vi "cast_to_32_bit.vi"(8 "input valid":bool=TRUE, 11 "x":fxp<+/-,64,48>) -> (0 "output valid":bool, 3 "y":fxp<+/-,32,14>)   [LabVIEW 2018]
uses:
  <vilib>/rvi/FXPMathLib/FxpConvert/subVIs/nifxpmath_Convert_SimConfig.ctl
  <vilib>/fxp/LVFixedPointQuantizationPolicyTypeDef.ctl
  <vilib>/fxp/LVFixedPointOverflowPolicyTypeDef.ctl
  <vilib>/rvi/FXPMathLib/FxpConvert/simVIs/DllFxpConvertTemp_sub.vi
  <vilib>/rvi/FXPMathLib/FxpInterpret/XNode/nifxpmath_Interpret.xnode
  <vilib>/rvi/FXPMathLib/FxpConvert/XNode/nifxpmath_Convert.xnode
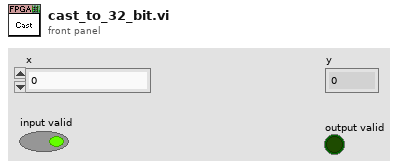
[diagram p1: front panel]
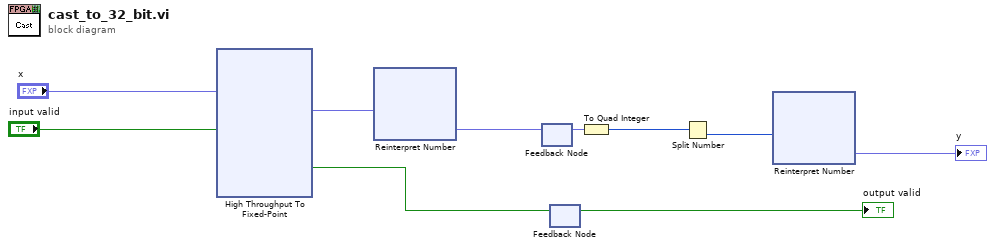
[diagram p0: block diagram]
diagram:
  n1 = xnode "High Throughput To Fixed-Point"("x"="x", "input valid"="input valid") -> ("y"=w9:fxp<+/-,64,56>, "output valid"=w2:bool)  [unwired: 1 in, 1 out]
  n2 = xnode "Reinterpret Number"("x"=w9) -> ("y"=w7:fxp<+/-,64,64>)
  n3 = feedback #1() -> (w4:fxp<+/-,64,64>)  [unwired: 1 in]
  n4 = feedback-in #1(w7) -> ()
  n5 = feedback #2() -> (→"output valid":bool)  [unwired: 1 in]
  n6 = feedback-in #2(w2) -> ()
  n7 = To Quad Integer(1:w4) -> (0:w8:i64)
  n8 = Split Number(x=w8) -> (lo(x)=w6:u32)  [unwired: 1 out]
  n9 = xnode "Reinterpret Number"("x"=w6) -> ("y"=→"y":fxp<+/-,32,14>)
